vi "Test_TextFileSink_FileSizeOverflow_NewFileCreated.vi"(8 "error in (no error)":errorcluster, 11 "TestCase in":refnum<class "TestTextFileSink.lvclass">) -> (0 "error out":errorcluster, 3 "TestCase out":refnum<class "TestTextFileSink.lvclass">)   [LabVIEW 2017, in "TestTextFileSink.lvclass"]
uses:
  TestTextFileSink.lvclass
  Source/Text File Sink/Configuration.ctl
  Source/Composed Log/LoggerReference/LoggerReference.lvclass/LoggerReference.ctl
  e024c6b3-4803-40b0-907f-2d7f922acde5.vi
  Source/Composed Log/LoggerReference/Return Aggregate Queues.vi
  Source/Composed Log/LoggerReference/Add Aggregate Log.vi
  e024c6b3-4803-40b0-907f-2d7f922acde5.vi/f37fe61c-6c11-44f8-b084-989469b2935e.vi
  Source/Composed Log/LoggerReference/Log.vi
  Source/Composed Log/LoggerReference/Send Add Sink.vi
  Source/Composed Log/LoggerReference/Remove Stale Logs.vi
  Source/Text File Sink/Text File Sink.lvclass
  C:/CS/Internal/LabVIEW/Logger/Source/Composed Log/Log Sink/Log Sink.lvclass
  Source/Composed Log/Application Logger/Launch Worker Loop.vi
  Source/Composed Log/LoggerReference/Initialize Logger Instance.vi
  Source/Composed Log/LoggerReference/LoggerReference.lvclass
  Source/Composed Log/IErrorFormat/IErrorFormat.lvclass
  Source/Composed Log/Log Sink/Log Sink.lvclass
  <vilib>/addons/_JKI Toolkits/VI Tester/TestCase.llb/TestCase.lvclass
  C:/Program Files (x86)/National Instruments/LabVIEW 2017/vi.lib/addons/_JKI Toolkits/VI Tester/TestCase.llb/TestCase.lvclass
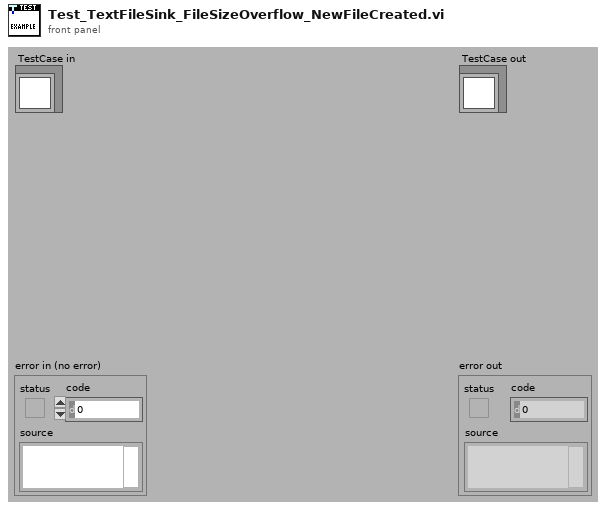
[diagram p1: front panel]
types:
  T1 = typedef "Text File Sink.lvclass/Configuration.ctl" = cluster{"Folder":path, "Name":string, "Extension":string, "Max Size (MB)":i64, "Timestamp Filename":bool}
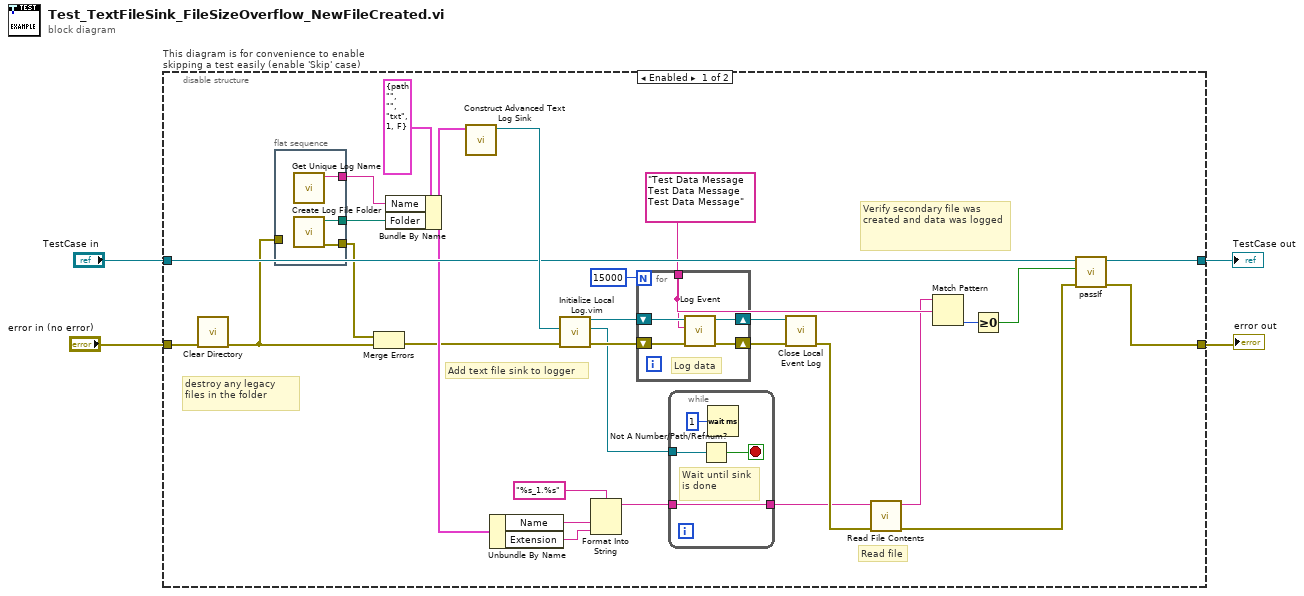
[diagram p0: block diagram]
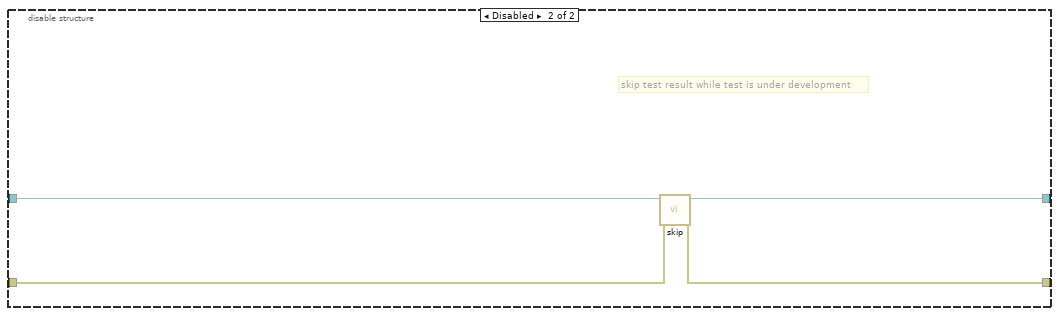
[diagram p2: hidden frame]
diagram:
  n1 = disable-structure "This diagram is for convenience to enable skipping a test easily (enable 'Skip' case)" shown="Enabled" {
    disable-tunnel: "TestCase in" -> [w25 w49]
    disable-tunnel: [w24 w47] -> w1
    disable-tunnel: [w22 w48] -> w3
    disable-tunnel: "error in (no error)" -> [w13 w46]
    frame Enabled {
      w11 = "Test Data Message Test Data Message Test Data Message" ("SourceID")
      # "destroy any legacy files in the folder"
      # "Read file"
      # "Verify secondary file was created and data was logged"
      # "Add text file sink to logger"
      n2 = call "Clear Directory.vi"("error in"=w13) -> ("error out"=w12:errorcluster)  [unwired: 10 in]
      n3 = flat-sequence {
        tunnel: [w40] -> w32
        tunnel: [w39] -> w16
        tunnel: [w38] -> w15
        tunnel: w12 -> [_]
        frame #0 {
          n4 = call "Get Unique Log Name.vi"() -> ("Log File Name"=w38:string)  [unwired: 11 in]
          n5 = call "Create Log File Folder.vi"() -> ("error out"=w39:errorcluster, "Folder Path"=w40:path)  [unwired: 10 in]
        }
      }
      n6 = Merge Errors(w16, w12) -> (w17:errorcluster)
      n7 = Bundle By Name(cluster=T1 {"Folder"=path "", "Name"="", "Extension"="txt", "Max Size (MB)"=1, "Timestamp Filename"=FALSE} ("Text File Configuration"), "Name"=w15, "Folder"=w32) -> (w21:T1)
      n8 = call "Construct Advanced Text Log Sink.vi"("Text File Configuration"=w21) -> ("Text File Sink out"=w31:refnum<class "Text File Sink.lvclass">)  [unwired: 10 in]
      n9 = Unbundle By Name(w21) -> ("Name"=w19:string, "Extension"=w18:string)
      n10 = call "Initialize Local Log.vim"("error in (no error)"=w17, "Startup Sink(s)"=w31) -> ("error out"=w30:errorcluster, "Log Sink Reference(s)"=w7:refnum<data-value>, "Log Instance Reference"=w29:refnum<class "LoggerReference.lvclass">)  [unwired: 7 in]
      n11 = Format Into String(format string="%s_1.%s", w19, w18) -> (resulting string=w6:string)  [unwired: 2 in, 1 out]
      n12 = for {
        N: 15000 -> [_]
        shift-right: [w43] -> w28
        shift-left: w30 -> [w45]
        shift-right: [w42] -> w27
        shift-left: w29 -> [w44]
        tunnel: w11 -> [w41]
        # "Log data"
        n13 = call "Log Event.vi"("error in (no error)"=w45, "SourceID"=w41, "Log Instance"=w44) -> ("error out"=w43:errorcluster, "Log Instance Out"=w42:refnum<class "LoggerReference.lvclass">)  [unwired: 7 in]
      }
      n14 = while {
        tunnel: w7 -> [w37]
        tunnel: w6 -> [w34]
        tunnel: [w34] -> w5
        stop <- w35 stop-if-true
        # "Wait until sink is done"
        n15 = Not A Number/Path/Refnum?(number/path/refnum=w37) -> (NaN/Path/Refnum?=w35:bool)
        n16 = Wait (ms)(milliseconds to wait=u32 1) -> ()  [unwired: 1 out]
      }
      n17 = call "Close Local Event Log.vi"("error in (no error)"=w28, "Log Instance"=w27) -> ("error out"=w26:errorcluster)  [unwired: 9 in]
      n18 = call "Read File Contents.vi"("error in (no error)"=w26, "File Name"=w5) -> ("error out"=w23:errorcluster, "File Text"=w10:string)  [unwired: 8 in]
      n19 = Match Pattern(string=w10, regular expression=w11) -> (offset past match=w9:i32)  [unwired: 1 in, 3 out]
      n20 = Greater Or Equal To 0?(x=w9) -> (x >= 0?=w8:bool)
      n21 = call-dynamic "passIf.vi"("error in (no error)"=w23, "pass"=w8, "TestCase in"=w25) -> ("error out"=w22:errorcluster, "TestCase out"=w24:refnum<class "TestTextFileSink.lvclass">)  [unwired: 7 in]
    }
    frame Disabled {
      # "skip test result while test is under development"
      n22 = call <vilib>:"skip.vi"("error in (no error)"=w46, "TestCase in"=w49) -> ("error out"=w48:errorcluster, "TestCase out"=w47:refnum<class "TestTextFileSink.lvclass">)  [unwired: 8 in]
    }
  }
  "error out" <- w3
  "TestCase out" <- w1
